vi "Core Energize.vi"(8 "error in (no error)":errorcluster, 11 "CIFCorePlugin in":refnum<class "CIFCorePlugin.lvclass">) -> (0 "error out":errorcluster, 3 "CIFCorePlugin out":refnum<class "CIFCorePlugin.lvclass">)   [LabVIEW 2021, in "CIFCorePlugin.lvclass"]
uses:
  CIFCorePlugin.lvclass
  CIFCorePlugin.lvclass/CIFCorePlugin.ctl
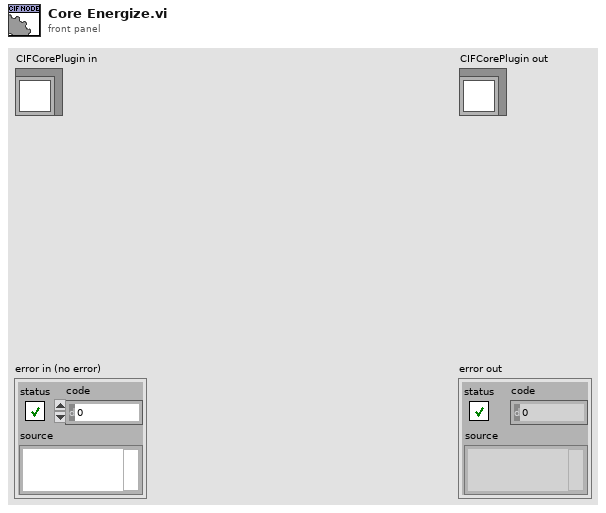
[diagram p1: front panel]
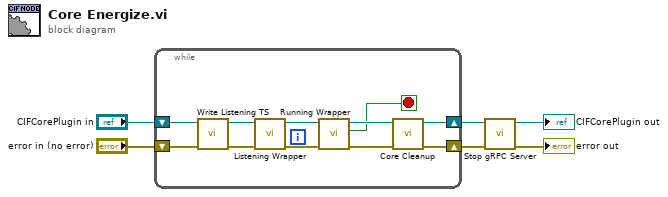
[diagram p0: block diagram]
diagram:
  n1 = while {
    shift-right: [w17] -> w3
    shift-left: "CIFCorePlugin in" -> [w15]
    shift-right: [w16] -> w2
    shift-left: "error in (no error)" -> [w14]
    stop <- w11 stop-if-true
    n2 = call "Write Listening TS.vi"("error in (no error)"=w14, "CIFCorePlugin in"=w15) -> ("error out"=w9:errorcluster, "CIFCorePlugin out"=w10:refnum<class "CIFCorePlugin.lvclass">)  [unwired: 8 in]
    n3 = call "Listening Wrapper.vi"("error in (no error)"=w9, "CIFCorePlugin in"=w10) -> ("error out"=w7:errorcluster, "CIFCorePlugin out"=w8:refnum<class "CIFCorePlugin.lvclass">)  [unwired: 8 in]
    n4 = call-dynamic "Running Wrapper.vi"("error in (no error)"=w7, "CIFCorePlugin in"=w8) -> ("error out"=w12:errorcluster, "Destroy"=w11:bool, "CIFCorePlugin out"=w13:refnum<class "CIFCorePlugin.lvclass">)  [unwired: 7 in]
    n5 = call "Core Cleanup.vi"("error in (no error)"=w12, "CIFTemplateNode in"=w13) -> ("error out"=w16:errorcluster, "CIFTemplateNode out"=w17:refnum<class "CIFCorePlugin.lvclass">)  [unwired: 8 in]
  }
  n6 = call "Stop gRPC Server.vi"("error in (no error)"=w2, "CIFCorePlugin in"=w3) -> ("error out"=→"error out":errorcluster, "CIFCorePlugin out"=→"CIFCorePlugin out":refnum<class "CIFCorePlugin.lvclass">)  [unwired: 8 in]
